vi "ResumeAutoTest.vi"(8 "error in (no error)":errorcluster, 11 "ExecutionControls in":refnum<class "ExecutionControls.lvclass">) -> (0 "error out":errorcluster, 3 "ExecutionControls out":refnum<class "ExecutionControls.lvclass">)   [LabVIEW 2018, in "ExecutionControls.lvclass"]
uses:
  ExecutionControls.lvclass
  <vilib>/Utility/miscctls.llb/LVForegroundBackgroundColorsTypeDef.ctl
  ExecutionControls.lvclass/ExecutionControls.ctl
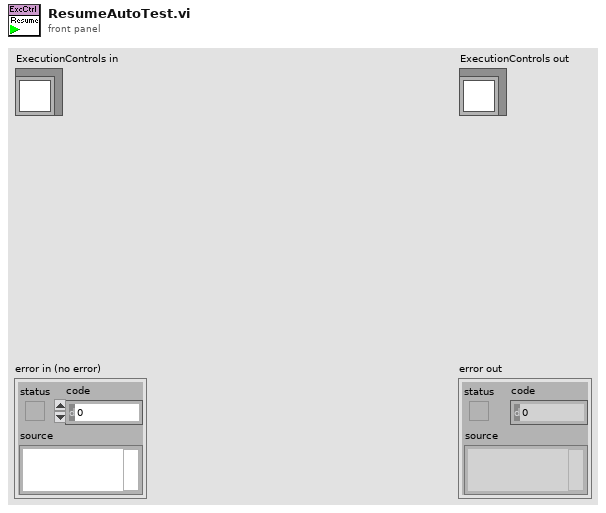
[diagram p1: front panel]
types:
  T1 = enum32{"Page Enabled", "Page Disabled", "Page Disabled & Grayed"}
  T2 = enum8{"Enabled", "Disabled", "Disabled and Grayed Out"}
  T3 = typedef "LVForegroundBackgroundColorsTypeDef.ctl" = cluster{"Foreground Color":u32, "Background Color":u32}
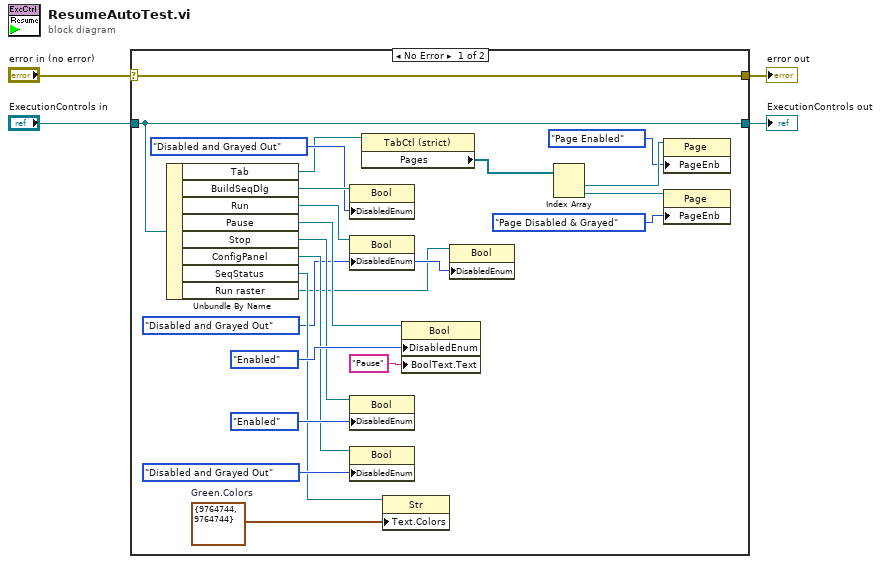
[diagram p0: block diagram]
diagram:
  n1 = case shown="No Error" "error in (no error)" {
    selector: "error in (no error)" -> [w26 w28]
    tunnel: [w26 w28] -> w1
    tunnel: [w16 w27] -> w2
    tunnel: "ExecutionControls in" -> [w16 w27]
    frame No Error {
      w7 = T3 {"Foreground Color"=9764744, "Background Color"=9764744}  # Green.Colors
      w6 = T2."Disabled and Grayed Out" ("Disabled")
      n2 = Unbundle By Name(w16) -> ("Tab"=w15:refnum<vi>, "BuildSeqDlg"=w25:refnum<vi>, "Run"=w23:refnum<vi>, "Pause"=w19:refnum<vi>, "Stop"=w18:refnum<vi>, "ConfigPanel"=w17:refnum<vi>, "SeqStatus"=w8:refnum<vi>, "Run raster"=w5:refnum<vi>)
      n3 = property class="Bool"(reference=w25, "DisabledEnum"=T2."Disabled and Grayed Out" ("Disabled")) -> ()  [unwired: 1 in, 2 out]
      n4 = property class="Bool"(reference=w23, "DisabledEnum"=w6) -> ()  [unwired: 1 in, 2 out]
      n5 = property class="Bool"(reference=w18, "DisabledEnum"=T2."Enabled" ("Disabled")) -> ()  [unwired: 1 in, 2 out]
      n6 = property class="Bool"(reference=w17, "DisabledEnum"=T2."Disabled and Grayed Out" ("Disabled")) -> ()  [unwired: 1 in, 2 out]
      n7 = property class="TabCtl (strict)"(reference=w15) -> ("Pages"=w14:refnum<vi>[])  [unwired: 1 in, 2 out]
      n8 = property class="Str"(reference=w8, "Text.Colors"=w7) -> ()  [unwired: 1 in, 2 out]
      n9 = property class="Bool"(reference=w19, "DisabledEnum"=T2."Enabled" ("Disabled"), "BoolText.Text"="Pause" ("Boolean Text.Text")) -> ()  [unwired: 1 in, 2 out]
      n10 = property class="Bool"(reference=w5, "DisabledEnum"=w6) -> ()  [unwired: 1 in, 2 out]
      n11 = Index Array(array=w14) -> (element #1=w12:refnum<vi>, element #2=w13:refnum<vi>)  [unwired: 2 in]
      n12 = property class="Page"(reference=w12, "PageEnb"=T1."Page Enabled" ("Page Enabled State")) -> ()  [unwired: 1 in, 2 out]
      n13 = property class="Page"(reference=w13, "PageEnb"=T1."Page Disabled & Grayed" ("Page Enabled State")) -> ()  [unwired: 1 in, 2 out]
    }
    frame Error {
    }
  }
  "error out" <- w1
  "ExecutionControls out" <- w2
